vi "Lockin.DAQ.TimedLoop.vi"(8 "error in (no error)":errorcluster, 10 "Event Cluster":T1, 11 "Lockin.DAQ in":refnum<class "Instrument.DAQ.lvclass">) -> (0 "error out":errorcluster, 3 "Lockin.DAQ out":refnum<class "Instrument.DAQ.lvclass">)   [LabVIEW 2019, in "Instrument.DAQ.lvclass"]
uses:
  Instrument.DAQ.lvclass
  C:/Program Files (x86)/National Instruments/LabVIEW 2019/vi.lib/JKI/JKI SMO/SMO/SMO.lvclass
  <vilib>/JKI/JKI SMO/SMO/Typedefs/Protected Events.ctl
  <vilib>/JKI/JKI SMO/SMO/Typedefs/StopProcessEventData--Cluster.ctl
  <vilib>/JKI/JKI SMO/SMO/Typedefs/AbortProcessEventData--Cluster.ctl
  <vilib>/JKI/JKI SMO/SMO/Typedefs/SMO Dependency Event--Cluster.ctl
  <vilib>/JKI/JKI SMO/SMO/Typedefs/SMO Dependency Event--Enum.ctl
  Typedefs/PrivateEvents--Cluster.ctl
  Typedefs/PrivateEvents--DAQ.setAOconfig.ctl
  Typedefs/AO.config-array.ctl
  Typedefs/AO.config-cluster.ctl
  Typedefs/446xAO-enum.ctl
  Typedefs/DAQType-enum.ctl
  Typedefs/PrivateEvents--DAQ.setAIconfig.ctl
  Typedefs/AI.config-array.ctl
  Typedefs/AI.config-cluster.ctl
  Typedefs/AI.coupling-enum.ctl
  Typedefs/446xAI-enum.ctl
  Typedefs/AI Simulation-enum.ctl
  Typedefs/PrivateEvents--DAQ.setAO.ctl
  Typedefs/AO-cluster.ctl
  Instrument UI.Lockin/Typedefs/AO Channel--Cluster.ctl
  Typedefs/Function-enum.ctl
  Typedefs/PrivateEvents--DAQ.setREF.ctl
  Typedefs/REF-cluster.ctl
  Instrument UI.Lockin/Typedefs/REF Channel--Cluster.ctl
  Typedefs/PrivateEvents--DAQ.setSampling.ctl
  Typedefs/Sampling.ctl
  Typedefs/Sample Mode--Ring.ctl
  Typedefs/PrivateEvents--DAQ.setState.ctl
  Typedefs/Set State-enum.ctl
  Typedefs/PrivateEvents--DAQ.setInputGain.ctl
  Typedefs/PrivateEvents--DAQ.setSweep.ctl
  Typedefs/Sweep Configuration--Cluster.ctl
  Instrument UI.Lockin/Typedefs/Sweep Channel--Cluster.ctl
  Typedefs/Sweep Pattern--Enum.ctl
  Typedefs/PrivateEvents--DAQ.measureOffset.ctl
  Typedefs/PrivateEvents--DAQ.zeroOffset.ctl
  Typedefs/PrivateEvents--DAQ.setPreFilter.ctl
  Typedefs/AI Prefilter-cluster.ctl
  Typedefs/PrivateEvents--DAQ.autoConfigureDAQ.ctl
  Typedefs/PrivateEvents--DAQ.setCalibration.ctl
  Typedefs/PrivateEvents--DAQ.setAI.ctl
  Typedefs/AI-cluster.ctl
  Instrument UI.Lockin/Typedefs/AI Channel--Cluster.ctl
  Typedefs/PrivateEvents--Lockin.DAQ.Reset Phase.ctl
  <vilib>/JKI/JKI SMO/SMO/SMO.lvclass/SMO.ctl
  Instrument.DAQ.lvclass/Instrument.DAQ.ctl
  <vilib>/Platform/TimedLoop/XDataNode/timing_clust.ctl
  <vilib>/Platform/TimedLoop/XDataNode/nitl_modes.ctl
  <vilib>/Platform/TimedLoop/XDataNode/wakeup.ctl
  <vilib>/JKI/JKI SMO/SMO/Private/ReftoDVR--SMO.vi
  <vilib>/platform/TimedLoop/XDataNode/XDataNode.xnode
  <vilib>/Platform/TimedLoop/XDataNode/XDNodeRunTimeDep.lvlib
  <vilib>/JKI/JKI SMO/SMO/SMO.lvclass
  Instrument UI.Lockin/Instrument UI.Lockin.lvclass
panel:
  out "Lockin":u32
  out "AO/AI":u32
  out "generate":u32
  # "!!!!!!!!!!!!!!!!!!!!!!!!!!!!!!!!!!!!!!!!!!!!!!!!!!!!!!!!!!!!!!!!!!!!!!!!\nTHIS IS AN EXPERIMENTAL BLOCKING CALL TO:\nGenerate\nRead/Write\nDSP\nIt should listen to events that change AO or REF Channels.\nInside there is a timed loop that will not stop unless it receives events for Set State = stop; SMO Stop; or SMO error\n!!!!!!!!!!!!!!!!!!!!!!!!!!!!!!!!!!!!!!!!!!!!!!!!!!!!!!!!!!!!!!!!!!!!!"
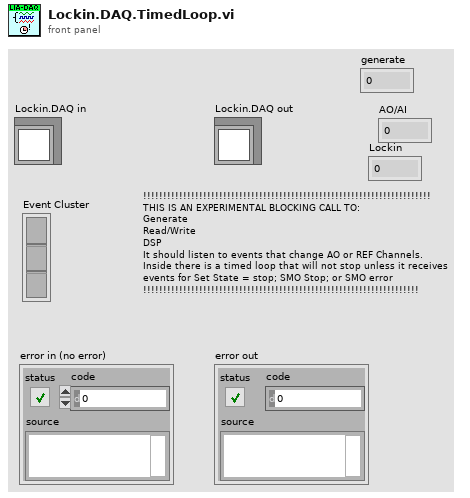
[diagram p1: front panel]
types:
  T1 = cluster{"SMO":refnum<event-registration>, "LockinDAQ":refnum<event-registration>, "DAQmx":refnum<event-registration>}
  T2 = typedef "SMO.lvclass/Protected Events.ctl" = cluster{"StopProcesses":refnum<user-event>, "AbortProcesses":refnum<user-event>, "Config Changed":refnum<user-event>, "Dependency":refnum<user-event>}
  T3 = typedef "Instrument.DAQ.lvclass/PrivateEvents--Cluster.ctl" = cluster{"setAOconfig":refnum<user-event>, "setAIconfig":refnum<user-event>, "setAO":refnum<user-event>, "setREF":refnum<user-event>, "setSampling":refnum<user-event>, "setState":refnum<user-event>, "setInputGain":refnum<user-event>, "setOutputGain":refnum<user-event>, "setSweep":refnum<user-event>, "measureOffset":refnum<user-event>, "zeroOffset":refnum<user-event>, "setPreFilter":refnum<user-event>, "autoConfigureDAQ":refnum<user-event>, "setCalibration":refnum<user-event>, "setAI":refnum<user-event>, "Reset Phase":refnum<user-event>}
  T4 = cluster{"Event Registration Refnum":refnum<event-registration>, "Event Registration Refnum":refnum<event-registration>}
  T5 = typedef "Instrument.DAQ.lvclass/Set State-enum.ctl" = enum16{"start", "stop", "reset", "start sweep", "stop sweep"}
  T6 = typedef "XDNodeRunTimeDep.lvlib/timing_clust.ctl" = cluster{"Expected End [f-1]":u64, "Actual End [f-1]":u64, "Finished Late? [f-1]":bool, "Expected End [i-1]":u64, "Actual End [i-1]":u64, "Finished Late? [i-1]":bool, "Expected Start [i]":u64, "Actual Start [i]":u64, "Expected Start [f]":u64, "Actual Start [f]":u64, "Source Name":string, "Structure Name":string, "Period":i64, "Deadline":i64, "Offset":i64, "Start":i64, "Priority":i32, "Timeout":i32, "Mode":T7, "Wakeup Reason":T8, "Error":errorcluster, "Source Type":string, "Secondary Source Type":string, "Global End Time":u64, "Global Start Time":u64, "Frame Duration":u64, "Iteration Duration":u64, "Assigned CPU":i32, "I/O Scan Engine Mode":u32}
  T7 = typedef "XDNodeRunTimeDep.lvlib/nitl_modes.ctl" = enum32{"No Change", "Process missed periods, maintain original phase", "Discard missed periods, maintain original phase", "Process missed periods, ignore original phase", "Discard missed periods, ignore original phase"}
  T8 = typedef "XDNodeRunTimeDep.lvlib/wakeup.ctl" = enum32{"Normal", "Aborted", "Asynchronous wakeup", "Timing source error", "Timed loop error", "Timeout"}
  T9 = cluster{"X":waveform(dbl)[], "Y":waveform(dbl)[]}
  T10 = typedef "Instrument.DAQ.lvclass/Results--Cluster.ctl" = cluster{"Time Stamp":timestamp, "Results (Dictionary)":cluster{"key":string, "value":dbl}[]}
  T11 = typedef "Instrument.DAQ.lvclass/AO-cluster.ctl" = T12[]
  T12 = typedef "Instrument UI.Lockin.lvclass/AO Channel--Cluster.ctl" = cluster{"Enable?":bool, "Channel":i32, "Amplitude":dbl, "Offset":dbl, "Frequency":dbl, "Phase":dbl, "Function":T13, "Sweeping?":bool}
  T13 = typedef "Instrument.DAQ.lvclass/Function-enum.ctl" = enum16{"Sine", "Triangle", "Square"}
  T14 = typedef "Instrument.DAQ.lvclass/REF-cluster.ctl" = T15[]
  T15 = typedef "Instrument UI.Lockin.lvclass/REF Channel--Cluster.ctl" = cluster{"Enable?":bool, "Channel":i32, "Frequency":dbl, "Phase":dbl, "TC":dbl, "Roll-Off":i32}
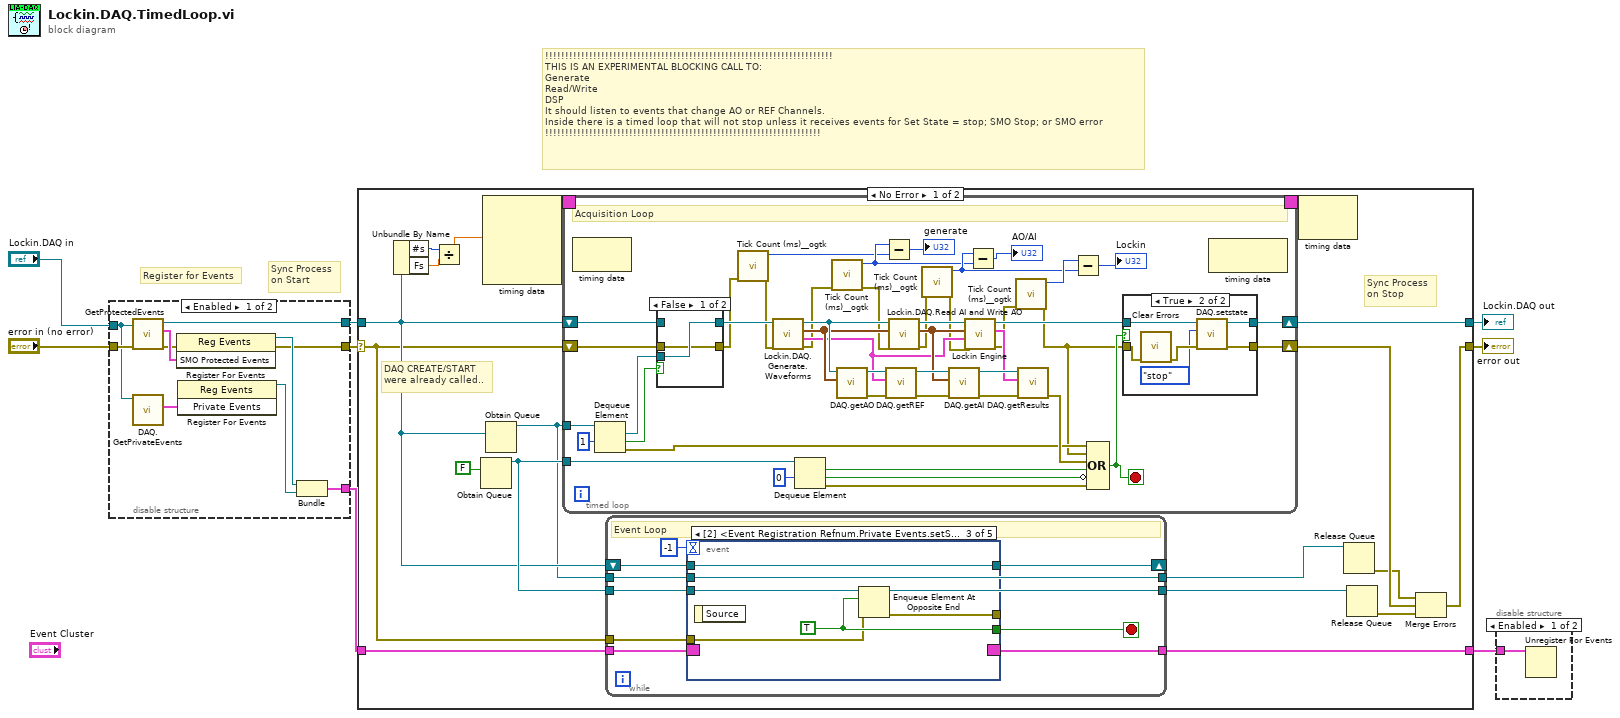
[diagram p0: block diagram]
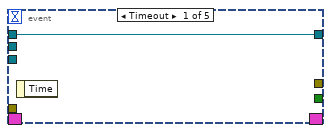
[diagram p6: hidden frame]
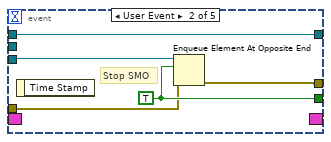
[diagram p7: hidden frame]
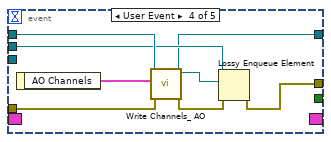
[diagram p8: hidden frame]
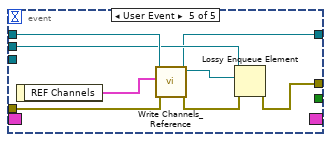
[diagram p9: hidden frame]
diagram:
  # "!!!!!!!!!!!!!!!!!!!!!!!!!!!!!!!!!!!!!!!!!!!!!!!!!!!!!!!!!!!!!!!!!!!!!!!!\nTHIS IS AN EXPERIMENTAL BLOCKING CALL TO:\nGenerate\nRead/Write\nDSP\nIt should listen to events that change AO or REF Channels.\nInside there is a timed loop that will not stop unless it receives events for Set State = stop; SMO Stop; or SMO error\n!!!!!!!!!!!!!!!!!!!!!!!!!!!!!!!!!!!!!!!!!!!!!!!!!!!!!!!!!!!!!!!!!!!!!"
  # "Sync Process\non Start"
  # "Register for Events"
  n1 = disable-structure shown="Enabled" {
    disable-tunnel: [w16 w20] -> w8
    disable-tunnel: "Lockin.DAQ in" -> [w9 w20]
    disable-tunnel: [w12 w19] -> w5
    disable-tunnel: "error in (no error)" -> [w11 w19]
    disable-tunnel: [w10 _] -> w3
    frame Enabled {
      n2 = call <vilib>:"GetProtectedEvents.vi"("error in (no error)"=w11, "SMO"=w9) -> ("error out"=w17:errorcluster, "SMO Protected Events"=w18:T2, "SMO out"=w16:refnum<class "Instrument.DAQ.lvclass">)  [unwired: 7 in]
      n3 = call "DAQ.GetPrivateEvents.vi"("Lockin.DAQ"=w9) -> ("Private Events"=w14:T3)  [unwired: 8 in, 2 out]
      n4 = register-events(error in=w17, w18) -> (reference out=w15:refnum<event-registration>, error out=w12:errorcluster)  [unwired: 1 in]
      n5 = register-events(w14) -> (reference out=w13:refnum<event-registration>)  [unwired: 2 in, 1 out]
      n6 = Bundle("Event Registration Refnum"=w15, "Event Registration Refnum"=w13) -> (w10:T4)  [unwired: 1 in]
    }
    frame Disabled {
    }
  }
  n7 = case shown="No Error" w5 {
    selector: w5 -> [w25 w137]
    tunnel: w8 -> [w26 w138]
    tunnel: w3 -> [w37 w139]
    tunnel: [w31 w137] -> w7
    tunnel: [w36 w139] -> w2
    tunnel: [w22 w138] -> w6
    frame No Error {
      # "DAQ CREATE/START\nwere already called.."
      # "Sync Process\non Stop"
      n8 = Unbundle By Name(w26) -> ("#s"=w30:i32, "Fs"=w28:dbl)
      n9 = Divide(x=w30, y=w28) -> (x/y=w29:dbl)
      n10 = Obtain Queue(element data type=FALSE) -> (queue out=w34:refnum<queue>)  [unwired: 4 in, 2 out]
      n11 = node-c288(w29) -> (w39:T6)  [unwired: 3 in]
      n12 = Obtain Queue(element data type=w26) -> (queue out=w21:refnum<queue>)  [unwired: 4 in, 2 out]
      n13 = timed-loop {
        timing: w39 -> [_]
        timing-out: [_] -> w38
        tunnel: w34 -> [w84]
        shift-right: [w56] -> w22
        shift-left: w26 -> [w61]
        shift-right: [w55] -> w27
        shift-left: w25 -> [w60]
        tunnel: w21 -> [w66]
        stop <- w58 stop-if-true
        # "Acquisition Loop"
        n14 = node-c288() -> ()  [unwired: 1 in, 1 out]
        n15 = Dequeue Element(queue=w66, timeout in ms (-1)=1) -> (element=w63:refnum<class "Instrument.DAQ.lvclass">, timed out?=w64:bool, error out=w59:errorcluster)  [unwired: 1 in, 1 out]
        n16 = case shown="False" w64 {
          tunnel: w63 -> [w94 _]
          tunnel: [w94 w96] -> w62
          tunnel: w61 -> [_ w96]
          tunnel: w60 -> [w93 w95]
          tunnel: [w93 w95] -> w54
          frame False {
          }
          frame True {
          }
        }
        n17 = call <userlib>:"Tick Count (ms)__ogtk.vi"("error in (no error)"=w54) -> ("error out"=w53:errorcluster, "millisecond timer value"=w43:u32)  [unwired: 9 in]
        n18 = call "Lockin.DAQ.Generate.Waveforms.vi"("error in (no error)"=w53, "Lockin.DAQ"=w62) -> ("error out"=w52:errorcluster, "Reference"=w71:T9, "AO []"=w77:waveform(dbl)[], "Lockin.DAQ"=w78:refnum<class "Instrument.DAQ.lvclass">)  [unwired: 6 in]
        n19 = Dequeue Element(queue=w84, timeout in ms (-1)=0) -> (element=w82:bool, timed out?=w81:bool, error out=w80:errorcluster)  [unwired: 1 in, 1 out]
        n20 = call <userlib>:"Tick Count (ms)__ogtk.vi"("error in (no error)"=w52) -> ("error out"=w51:errorcluster, "millisecond timer value"=w44:u32)  [unwired: 9 in]
        n21 = call "DAQ.getAO.vi"("get AO"=w77, "Lockin.DAQ"=w78) -> ("error out"=w76:errorcluster, "Lockin.DAQ"=w79:refnum<class "Instrument.DAQ.lvclass">)  [unwired: 8 in]
        n22 = Subtract(x=w44, y=w43) -> (x-y=→"generate":u32)
        n23 = call "DAQ.getREF.vi"("error in (no error)"=w76, "getREF"=w71, "Lockin.DAQ"=w79) -> ("error out"=w75:errorcluster, "Lockin.DAQ"=w74:refnum<class "Instrument.DAQ.lvclass">)  [unwired: 7 in]
        n24 = call "Lockin.DAQ.Read AI and Write AO.vi"("error in (no error)"=w51, "AO []"=w77, "Lockin.DAQ in"=w78) -> ("error out"=w50:errorcluster, "AI []"=w73:waveform(dbl)[], "Lockin.DAQ out"=w72:refnum<class "Instrument.DAQ.lvclass">)  [unwired: 5 in, 1 out]
        n25 = call <userlib>:"Tick Count (ms)__ogtk.vi"("error in (no error)"=w50) -> ("error out"=w49:errorcluster, "millisecond timer value"=w45:u32)  [unwired: 9 in]
        n26 = call "DAQ.getAI.vi"("error in (no error)"=w75, "getAI"=w73, "Lockin.DAQ"=w74) -> ("error out"=w70:errorcluster, "Lockin.DAQ"=w69:refnum<class "Instrument.DAQ.lvclass">)  [unwired: 7 in]
        n27 = call "Lockin Engine.vi"("error in (no error)"=w49, "Reference"=w71, "AI Waveforms"=w73, "Lockin.DAQ"=w72) -> ("error out"=w48:errorcluster, "Averaged Results (X,Y,R,Theta,Mean)"=w68:T10, "Lockin.DAQ"=w57:refnum<class "Instrument.DAQ.lvclass">)  [unwired: 4 in, 1 out]
        n28 = Subtract(x=w45, y=w44) -> (x-y=→"AO/AI":u32)
        n29 = call <userlib>:"Tick Count (ms)__ogtk.vi"("error in (no error)"=w48) -> ("error out"=w47:errorcluster, "millisecond timer value"=w46:u32)  [unwired: 9 in]
        n30 = call "DAQ.getResults.vi"("error in (no error)"=w70, "Results"=w68, "Lockin.DAQ"=w69) -> ("error out"=w67:errorcluster)  [unwired: 7 in, 1 out]
        n31 = Subtract(x=w46, y=w45) -> (x-y=→"Lockin":u32)
        n32 = Compound Arithmetic op=OR(w59, w47, w67, w82, invert w81, w80) -> (w58:bool)
        n33 = case shown="True" w58 {
          tunnel: w57 -> [w85 w92]
          tunnel: [w85 w91] -> w56
          tunnel: [w86 w90] -> w55
          tunnel: w47 -> [w86 w88]
          frame False {
          }
          frame True {
            n34 = call <vilib>:"Clear Errors.vi"("error in (no error)"=w88) -> ("error out"=w89:errorcluster)  [unwired: 5 in, 1 out]
            n35 = call "DAQ.setstate.vi"("error in (no error)"=w89, "State"=Set_State-enum."stop" ("setState"), "Lockin.DAQ"=w92) -> ("error out"=w90:errorcluster, "Lockin.DAQ out"=w91:refnum<class "Instrument.DAQ.lvclass">)  [unwired: 7 in]
          }
        }
        n36 = node-c288() -> ()  [unwired: 1 in, 1 out]
      }
      n37 = while {
        tunnel: w37 -> [w109]
        tunnel: [w108] -> w36
        shift-right: [w105] -> _
        shift-left: w26 -> [w106]
        tunnel: w25 -> [w104]
        tunnel: w21 -> [w103]
        tunnel: [w103] -> w24
        tunnel: w34 -> [w102]
        tunnel: [w102] -> w33
        stop <- w107 stop-if-true
        # "Event Loop"
        n38 = event shown="[2] <Event Registration Refnum.Private Events.setState>: User Event" {
          selector: w109 -> [_ _ _ _ _]
          dyn-events: [_ _ _ _ _] -> w108
          timeout: -1 -> [_ _ _ _ _]
          tunnel: [_ w115 w118 _ _] -> w107
          tunnel: w102 -> [_ w116 w121 _ _]
          tunnel: [_ w112 w120 w122 w130] -> _
          tunnel: w106 -> [w111 w114 w119 w128 w135]
          tunnel: [w111 w114 w119 w124 w129] -> w105
          tunnel: w104 -> [_ w113 w117 w127 w133]
          tunnel: w103 -> [_ _ _ w125 w132]
          event Timeout {
            n39 = event-data() -> ()  [unwired: 1 in, 1 out]
          }
          event User Event {
            w115 = TRUE
            # "Stop SMO"
            n40 = event-data() -> ()  [unwired: 1 in, 1 out]
            n41 = Enqueue Element At Opposite End(queue=w116, element=w115, error in (no error)=w113) -> (error out=w112:errorcluster)  [unwired: 1 in, 2 out]
          }
          event User Event {
            w118 = TRUE
            n42 = event-data() -> ()  [unwired: 1 in, 1 out]
            n43 = Enqueue Element At Opposite End(queue=w121, element=w118, error in (no error)=w117) -> (error out=w120:errorcluster)  [unwired: 1 in, 2 out]
          }
          event User Event {
            n44 = event-data() -> ("AO Channels"=w126:T11)  [unwired: 1 in]
            n45 = call "Write Channels_ AO.vi"("error in (no error)"=w127, "Channels: AO"=w126, "Lockin.DAQ"=w128) -> ("error out"=w123:errorcluster, "Lockin.DAQ out"=w124:refnum<class "Instrument.DAQ.lvclass">)  [unwired: 7 in]
            n46 = Lossy Enqueue Element(queue=w125, element=w124, error in (no error)=w123) -> (error out=w122:errorcluster)  [unwired: 3 out]
          }
          event User Event {
            n47 = event-data() -> ("REF Channels"=w134:T14)  [unwired: 1 in]
            n48 = call "Write Channels_ Reference.vi"("error in (no error)"=w133, "Configuration.Channels: REF"=w134, "Lockin.DAQ"=w135) -> ("error out"=w131:errorcluster, "Lockin.DAQ out"=w129:refnum<class "Instrument.DAQ.lvclass">)  [unwired: 7 in]
            n49 = Lossy Enqueue Element(queue=w132, element=w129, error in (no error)=w131) -> (error out=w130:errorcluster)  [unwired: 3 out]
          }
        }
      }
      n50 = node-c288(w38) -> ()  [unwired: 1 out]
      n51 = Release Queue(queue=w24) -> (error out=w23:errorcluster)  [unwired: 2 in, 2 out]
      n52 = Release Queue(queue=w33) -> (error out=w32:errorcluster)  [unwired: 2 in, 2 out]
      n53 = Merge Errors(w23, w27, w32) -> (w31:errorcluster)
    }
    frame Error {
    }
  }
  "error out" <- w7
  "Lockin.DAQ out" <- w6
  n54 = disable-structure shown="Enabled" {
    disable-tunnel: w2 -> [w140 _]
    frame Enabled {
      n55 = Unregister For Events(event registration refnum=w140) -> ()  [unwired: 1 in, 1 out]
    }
    frame Disabled {
    }
  }
